vi "PiratiZKaribiku.vi"(11 "NXT/EV3":T1) -> (3 "NXT/EV3 2":T1)   [LabVIEW 2016]
uses:
  <vilib>/NXT/Subs/LVHSConnector.ctl
  <vilib>/NXT/LegoClasses/BrickReference/BrickReference.lvclass
  <vilib>/NXT/Dual Mode Library/Display/drawText_Center.vi
  <vilib>/NXT/Dual Mode Library/Sound/PlayA.vi
  <vilib>/NXT/Dual Mode Library/Sound/PlayC.vi
  <vilib>/NXT/Dual Mode Library/Sound/PlayD.vi
  <vilib>/NXT/Dual Mode Library/Sound/PlayE.vi
  <vilib>/NXT/Dual Mode Library/Sound/PlayF.vi
  <vilib>/NXT/Dual Mode Library/Sound/PlayG.vi
  <vilib>/NXT/Dual Mode Library/Waits/Wait_Num.vi
  <vilib>/NXT/Dual Mode Library/Sound/PlayB.vi
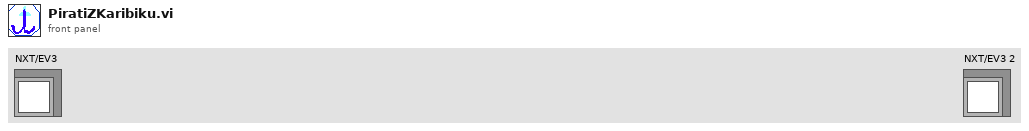
[diagram p1: front panel]
types:
  T1 = typedef "LVHSConnector.ctl" = refnum<class "BrickReference.lvclass">
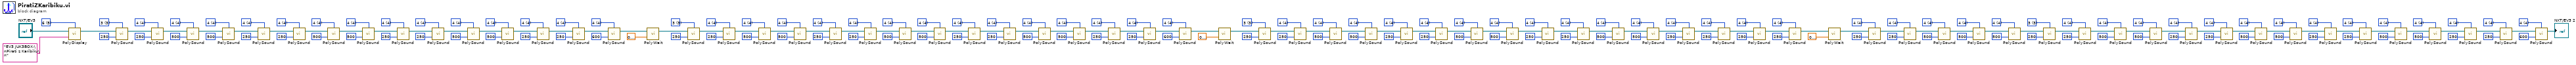
[diagram p0: block diagram]
diagram:
  w18 = u16 4 items=["3"=3, "4"=4, "5"=5, "6"=6, "7"=7] ("Octave")
  w21 = u16 4 items=["3"=3, "4"=4, "5"=5, "6"=6, "7"=7] ("Octave")
  w19 = u16 4 items=["3"=3, "4"=4, "5"=5, "6"=6, "7"=7] ("Octave")
  w26 = u16 4 items=["3"=3, "4"=4, "5"=5, "6"=6, "7"=7] ("Octave")
  w27 = u16 4 items=["3"=3, "4"=4, "5"=5, "6"=6, "7"=7] ("Octave")
  w28 = u16 4 items=["3"=3, "4"=4, "5"=5, "6"=6, "7"=7] ("Octave")
  w32 = u16 4 items=["3"=3, "4"=4, "5"=5, "6"=6, "7"=7] ("Octave")
  w33 = u16 4 items=["3"=3, "4"=4, "5"=5, "6"=6, "7"=7] ("Octave")
  w34 = u16 4 items=["3"=3, "4"=4, "5"=5, "6"=6, "7"=7] ("Octave")
  w36 = u16 4 items=["3"=3, "4"=4, "5"=5, "6"=6, "7"=7] ("Octave")
  w42 = u16 4 items=["3"=3, "4"=4, "5"=5, "6"=6, "7"=7] ("Octave")
  w43 = u16 4 items=["3"=3, "4"=4, "5"=5, "6"=6, "7"=7] ("Octave")
  w44 = u16 3 items=["3"=3, "4"=4, "5"=5, "6"=6, "7"=7] ("Octave")
  w45 = u16 4 items=["3"=3, "4"=4, "5"=5, "6"=6, "7"=7] ("Octave")
  w46 = u16 4 items=["3"=3, "4"=4, "5"=5, "6"=6, "7"=7] ("Octave")
  w49 = u16 4 items=["3"=3, "4"=4, "5"=5, "6"=6, "7"=7] ("Octave")
  w52 = u16 4 items=["3"=3, "4"=4, "5"=5, "6"=6, "7"=7] ("Octave")
  w55 = u16 4 items=["3"=3, "4"=4, "5"=5, "6"=6, "7"=7] ("Octave")
  w82 = u16 4 items=["3"=3, "4"=4, "5"=5, "6"=6, "7"=7] ("Octave")
  w83 = u16 4 items=["3"=3, "4"=4, "5"=5, "6"=6, "7"=7] ("Octave")
  w90 = u16 4 items=["3"=3, "4"=4, "5"=5, "6"=6, "7"=7] ("Octave")
  w89 = u16 4 items=["3"=3, "4"=4, "5"=5, "6"=6, "7"=7] ("Octave")
  w96 = u16 4 items=["3"=3, "4"=4, "5"=5, "6"=6, "7"=7] ("Octave")
  w97 = u16 4 items=["3"=3, "4"=4, "5"=5, "6"=6, "7"=7] ("Octave")
  w103 = u16 4 items=["3"=3, "4"=4, "5"=5, "6"=6, "7"=7] ("Octave")
  w100 = u16 4 items=["3"=3, "4"=4, "5"=5, "6"=6, "7"=7] ("Octave")
  w108 = u16 4 items=["3"=3, "4"=4, "5"=5, "6"=6, "7"=7] ("Octave")
  w107 = u16 4 items=["3"=3, "4"=4, "5"=5, "6"=6, "7"=7] ("Octave")
  w115 = u16 4 items=["3"=3, "4"=4, "5"=5, "6"=6, "7"=7] ("Octave")
  w119 = u16 4 items=["3"=3, "4"=4, "5"=5, "6"=6, "7"=7] ("Octave")
  w122 = u16 4 items=["3"=3, "4"=4, "5"=5, "6"=6, "7"=7] ("Octave")
  w129 = u16 4 items=["3"=3, "4"=4, "5"=5, "6"=6, "7"=7] ("Octave")
  w128 = u16 4 items=["3"=3, "4"=4, "5"=5, "6"=6, "7"=7] ("Octave")
  w127 = u16 3 items=["3"=3, "4"=4, "5"=5, "6"=6, "7"=7] ("Octave")
  w126 = u16 4 items=["3"=3, "4"=4, "5"=5, "6"=6, "7"=7] ("Octave")
  w125 = u16 4 items=["3"=3, "4"=4, "5"=5, "6"=6, "7"=7] ("Octave")
  w175 = u16 4 items=["3"=3, "4"=4, "5"=5, "6"=6, "7"=7] ("Octave")
  w169 = u16 4 items=["3"=3, "4"=4, "5"=5, "6"=6, "7"=7] ("Octave")
  w172 = u16 4 items=["3"=3, "4"=4, "5"=5, "6"=6, "7"=7] ("Octave")
  w164 = u16 4 items=["3"=3, "4"=4, "5"=5, "6"=6, "7"=7] ("Octave")
  w163 = u16 4 items=["3"=3, "4"=4, "5"=5, "6"=6, "7"=7] ("Octave")
  w162 = u16 4 items=["3"=3, "4"=4, "5"=5, "6"=6, "7"=7] ("Octave")
  w155 = u16 4 items=["3"=3, "4"=4, "5"=5, "6"=6, "7"=7] ("Octave")
  w154 = u16 4 items=["3"=3, "4"=4, "5"=5, "6"=6, "7"=7] ("Octave")
  w153 = u16 4 items=["3"=3, "4"=4, "5"=5, "6"=6, "7"=7] ("Octave")
  w150 = u16 4 items=["3"=3, "4"=4, "5"=5, "6"=6, "7"=7] ("Octave")
  w144 = u16 4 items=["3"=3, "4"=4, "5"=5, "6"=6, "7"=7] ("Octave")
  w143 = u16 4 items=["3"=3, "4"=4, "5"=5, "6"=6, "7"=7] ("Octave")
  w142 = u16 3 items=["3"=3, "4"=4, "5"=5, "6"=6, "7"=7] ("Octave")
  w141 = u16 4 items=["3"=3, "4"=4, "5"=5, "6"=6, "7"=7] ("Octave")
  w140 = u16 4 items=["3"=3, "4"=4, "5"=5, "6"=6, "7"=7] ("Octave")
  w178 = u16 4 items=["3"=3, "4"=4, "5"=5, "6"=6, "7"=7] ("Octave")
  w179 = i16 5 items=["1", "2", "3", "4", "5", "6", "7", "8", "9", "10", "11", "12"] ("Line")
  w183 = u16 4 items=["3"=3, "4"=4, "5"=5, "6"=6, "7"=7] ("Octave")
  w181 = u16 4 items=["3"=3, "4"=4, "5"=5, "6"=6, "7"=7] ("Octave")
  w188 = u16 4 items=["3"=3, "4"=4, "5"=5, "6"=6, "7"=7] ("Octave")
  w189 = u16 4 items=["3"=3, "4"=4, "5"=5, "6"=6, "7"=7] ("Octave")
  w190 = u16 4 items=["3"=3, "4"=4, "5"=5, "6"=6, "7"=7] ("Octave")
  w194 = u16 4 items=["3"=3, "4"=4, "5"=5, "6"=6, "7"=7] ("Octave")
  w195 = u16 4 items=["3"=3, "4"=4, "5"=5, "6"=6, "7"=7] ("Octave")
  w196 = u16 4 items=["3"=3, "4"=4, "5"=5, "6"=6, "7"=7] ("Octave")
  w198 = u16 4 items=["3"=3, "4"=4, "5"=5, "6"=6, "7"=7] ("Octave")
  w204 = u16 4 items=["3"=3, "4"=4, "5"=5, "6"=6, "7"=7] ("Octave")
  w205 = u16 4 items=["3"=3, "4"=4, "5"=5, "6"=6, "7"=7] ("Octave")
  w206 = u16 3 items=["3"=3, "4"=4, "5"=5, "6"=6, "7"=7] ("Octave")
  w207 = u16 4 items=["3"=3, "4"=4, "5"=5, "6"=6, "7"=7] ("Octave")
  w208 = u16 4 items=["3"=3, "4"=4, "5"=5, "6"=6, "7"=7] ("Octave")
  n1 = call-poly <vilib>:"PolyDisplay.vi"("Text"="EV3 JUK3BOX:\nPirati z Karibiku\n", "NXT/EV3"="NXT/EV3", "Line"=w179) -> ("NXT/EV3"=w78:T1)  [unwired: 1 in]
  n2 = call-poly <vilib>:"PolySound.vi"("Duration (500 ms)"=u16 250, "NXT/EV3"=w78, "Octave"=w206) -> ("NXT/EV3"=w77:T1)  [unwired: 1 in]
  n3 = call-poly <vilib>:"PolySound.vi"("Duration (500 ms)"=u16 250, "NXT/EV3"=w77, "Octave"=w208) -> ("NXT/EV3"=w76:T1)  [unwired: 1 in]
  n4 = call-poly <vilib>:"PolySound.vi"("Duration (500 ms)"=u16 500, "NXT/EV3"=w76, "Octave"=w207) -> ("NXT/EV3"=w75:T1)  [unwired: 1 in]
  n5 = call-poly <vilib>:"PolySound.vi"("Duration (500 ms)"=u16 500, "NXT/EV3"=w75, "Octave"=w205) -> ("NXT/EV3"=w74:T1)  [unwired: 1 in]
  n6 = call-poly <vilib>:"PolySound.vi"("Duration (500 ms)"=u16 250, "NXT/EV3"=w74, "Octave"=w204) -> ("NXT/EV3"=w73:T1)  [unwired: 1 in]
  n7 = call-poly <vilib>:"PolySound.vi"("Duration (500 ms)"=u16 250, "NXT/EV3"=w73, "Octave"=w198) -> ("NXT/EV3"=w72:T1)  [unwired: 1 in]
  n8 = call-poly <vilib>:"PolySound.vi"("Duration (500 ms)"=u16 500, "NXT/EV3"=w72, "Octave"=w196) -> ("NXT/EV3"=w71:T1)  [unwired: 1 in]
  n9 = call-poly <vilib>:"PolySound.vi"("Duration (500 ms)"=u16 500, "NXT/EV3"=w71, "Octave"=w195) -> ("NXT/EV3"=w70:T1)  [unwired: 1 in]
  n10 = call-poly <vilib>:"PolySound.vi"("Duration (500 ms)"=u16 250, "NXT/EV3"=w70, "Octave"=w194) -> ("NXT/EV3"=w69:T1)  [unwired: 1 in]
  n11 = call-poly <vilib>:"PolySound.vi"("Duration (500 ms)"=u16 250, "NXT/EV3"=w69, "Octave"=w190) -> ("NXT/EV3"=w68:T1)  [unwired: 1 in]
  n12 = call-poly <vilib>:"PolySound.vi"("Duration (500 ms)"=u16 500, "NXT/EV3"=w68, "Octave"=w188) -> ("NXT/EV3"=w67:T1)  [unwired: 1 in]
  n13 = call-poly <vilib>:"PolySound.vi"("Duration (500 ms)"=u16 500, "NXT/EV3"=w67, "Octave"=w189) -> ("NXT/EV3"=w66:T1)  [unwired: 1 in]
  n14 = call-poly <vilib>:"PolySound.vi"("Duration (500 ms)"=u16 250, "NXT/EV3"=w66, "Octave"=w181) -> ("NXT/EV3"=w65:T1)  [unwired: 1 in]
  n15 = call-poly <vilib>:"PolySound.vi"("Duration (500 ms)"=u16 250, "NXT/EV3"=w65, "Octave"=w183) -> ("NXT/EV3"=w64:T1)  [unwired: 1 in]
  n16 = call-poly <vilib>:"PolySound.vi"("Duration (500 ms)"=u16 600, "NXT/EV3"=w64, "Octave"=w178) -> ("NXT/EV3"=w63:T1)  [unwired: 1 in]
  n17 = call-poly <vilib>:"PolyWait.vi"("Time (1 sec)"=sgl 0.4, "NXT/EV3"=w63) -> ("NXT/EV3"=w139:T1)  [unwired: 2 in]
  n18 = call-poly <vilib>:"PolySound.vi"("Duration (500 ms)"=u16 250, "NXT/EV3"=w139, "Octave"=w142) -> ("NXT/EV3"=w62:T1)  [unwired: 1 in]
  n19 = call-poly <vilib>:"PolySound.vi"("Duration (500 ms)"=u16 250, "NXT/EV3"=w62, "Octave"=w140) -> ("NXT/EV3"=w61:T1)  [unwired: 1 in]
  n20 = call-poly <vilib>:"PolySound.vi"("Duration (500 ms)"=u16 500, "NXT/EV3"=w61, "Octave"=w141) -> ("NXT/EV3"=w60:T1)  [unwired: 1 in]
  n21 = call-poly <vilib>:"PolySound.vi"("Duration (500 ms)"=u16 500, "NXT/EV3"=w60, "Octave"=w143) -> ("NXT/EV3"=w59:T1)  [unwired: 1 in]
  n22 = call-poly <vilib>:"PolySound.vi"("Duration (500 ms)"=u16 250, "NXT/EV3"=w59, "Octave"=w144) -> ("NXT/EV3"=w58:T1)  [unwired: 1 in]
  n23 = call-poly <vilib>:"PolySound.vi"("Duration (500 ms)"=u16 250, "NXT/EV3"=w58, "Octave"=w150) -> ("NXT/EV3"=w57:T1)  [unwired: 1 in]
  n24 = call-poly <vilib>:"PolySound.vi"("Duration (500 ms)"=u16 500, "NXT/EV3"=w57, "Octave"=w153) -> ("NXT/EV3"=w56:T1)  [unwired: 1 in]
  n25 = call-poly <vilib>:"PolySound.vi"("Duration (500 ms)"=u16 500, "NXT/EV3"=w56, "Octave"=w154) -> ("NXT/EV3"=w152:T1)  [unwired: 1 in]
  n26 = call-poly <vilib>:"PolySound.vi"("Duration (500 ms)"=u16 250, "NXT/EV3"=w152, "Octave"=w155) -> ("NXT/EV3"=w159:T1)  [unwired: 1 in]
  n27 = call-poly <vilib>:"PolySound.vi"("Duration (500 ms)"=u16 250, "NXT/EV3"=w159, "Octave"=w162) -> ("NXT/EV3"=w160:T1)  [unwired: 1 in]
  n28 = call-poly <vilib>:"PolySound.vi"("Duration (500 ms)"=u16 500, "NXT/EV3"=w160, "Octave"=w164) -> ("NXT/EV3"=w161:T1)  [unwired: 1 in]
  n29 = call-poly <vilib>:"PolySound.vi"("Duration (500 ms)"=u16 500, "NXT/EV3"=w161, "Octave"=w163) -> ("NXT/EV3"=w173:T1)  [unwired: 1 in]
  n30 = call-poly <vilib>:"PolySound.vi"("Duration (500 ms)"=u16 250, "NXT/EV3"=w173, "Octave"=w172) -> ("NXT/EV3"=w170:T1)  [unwired: 1 in]
  n31 = call-poly <vilib>:"PolySound.vi"("Duration (500 ms)"=u16 250, "NXT/EV3"=w170, "Octave"=w169) -> ("NXT/EV3"=w174:T1)  [unwired: 1 in]
  n32 = call-poly <vilib>:"PolySound.vi"("Duration (500 ms)"=u16 600, "NXT/EV3"=w174, "Octave"=w175) -> ("NXT/EV3"=w112:T1)  [unwired: 1 in]
  n33 = call-poly <vilib>:"PolyWait.vi"("Time (1 sec)"=sgl 0.4, "NXT/EV3"=w112) -> ("NXT/EV3"=w111:T1)  [unwired: 2 in]
  n34 = call-poly <vilib>:"PolySound.vi"("Duration (500 ms)"=u16 250, "NXT/EV3"=w111, "Octave"=w127) -> ("NXT/EV3"=w131:T1)  [unwired: 1 in]
  n35 = call-poly <vilib>:"PolySound.vi"("Duration (500 ms)"=u16 250, "NXT/EV3"=w131, "Octave"=w125) -> ("NXT/EV3"=w123:T1)  [unwired: 1 in]
  n36 = call-poly <vilib>:"PolySound.vi"("Duration (500 ms)"=u16 500, "NXT/EV3"=w123, "Octave"=w126) -> ("NXT/EV3"=w130:T1)  [unwired: 1 in]
  n37 = call-poly <vilib>:"PolySound.vi"("Duration (500 ms)"=u16 500, "NXT/EV3"=w130, "Octave"=w128) -> ("NXT/EV3"=w124:T1)  [unwired: 1 in]
  n38 = call-poly <vilib>:"PolySound.vi"("Duration (500 ms)"=u16 250, "NXT/EV3"=w124, "Octave"=w129) -> ("NXT/EV3"=w120:T1)  [unwired: 1 in]
  n39 = call-poly <vilib>:"PolySound.vi"("Duration (500 ms)"=u16 250, "NXT/EV3"=w120, "Octave"=w122) -> ("NXT/EV3"=w117:T1)  [unwired: 1 in]
  n40 = call-poly <vilib>:"PolySound.vi"("Duration (500 ms)"=u16 500, "NXT/EV3"=w117, "Octave"=w119) -> ("NXT/EV3"=w114:T1)  [unwired: 1 in]
  n41 = call-poly <vilib>:"PolySound.vi"("Duration (500 ms)"=u16 500, "NXT/EV3"=w114, "Octave"=w115) -> ("NXT/EV3"=w105:T1)  [unwired: 1 in]
  n42 = call-poly <vilib>:"PolySound.vi"("Duration (500 ms)"=u16 250, "NXT/EV3"=w105, "Octave"=w107) -> ("NXT/EV3"=w110:T1)  [unwired: 1 in]
  n43 = call-poly <vilib>:"PolySound.vi"("Duration (500 ms)"=u16 250, "NXT/EV3"=w110, "Octave"=w108) -> ("NXT/EV3"=w99:T1)  [unwired: 1 in]
  n44 = call-poly <vilib>:"PolySound.vi"("Duration (500 ms)"=u16 500, "NXT/EV3"=w99, "Octave"=w100) -> ("NXT/EV3"=w104:T1)  [unwired: 1 in]
  n45 = call-poly <vilib>:"PolySound.vi"("Duration (500 ms)"=u16 500, "NXT/EV3"=w104, "Octave"=w103) -> ("NXT/EV3"=w93:T1)  [unwired: 1 in]
  n46 = call-poly <vilib>:"PolySound.vi"("Duration (500 ms)"=u16 250, "NXT/EV3"=w93, "Octave"=w97) -> ("NXT/EV3"=w94:T1)  [unwired: 1 in]
  n47 = call-poly <vilib>:"PolySound.vi"("Duration (500 ms)"=u16 250, "NXT/EV3"=w94, "Octave"=w96) -> ("NXT/EV3"=w87:T1)  [unwired: 1 in]
  n48 = call-poly <vilib>:"PolySound.vi"("Duration (500 ms)"=u16 250, "NXT/EV3"=w87, "Octave"=w89) -> ("NXT/EV3"=w92:T1)  [unwired: 1 in]
  n49 = call-poly <vilib>:"PolySound.vi"("Duration (500 ms)"=u16 250, "NXT/EV3"=w92, "Octave"=w90) -> ("NXT/EV3"=w86:T1)  [unwired: 1 in]
  n50 = call-poly <vilib>:"PolyWait.vi"("Time (1 sec)"=sgl 0.4, "NXT/EV3"=w86) -> ("NXT/EV3"=w79:T1)  [unwired: 2 in]
  n51 = call-poly <vilib>:"PolySound.vi"("Duration (500 ms)"=u16 250, "NXT/EV3"=w79, "Octave"=w83) -> ("NXT/EV3"=w80:T1)  [unwired: 1 in]
  n52 = call-poly <vilib>:"PolySound.vi"("Duration (500 ms)"=u16 250, "NXT/EV3"=w80, "Octave"=w82) -> ("NXT/EV3"=w50:T1)  [unwired: 1 in]
  n53 = call-poly <vilib>:"PolySound.vi"("Duration (500 ms)"=u16 500, "NXT/EV3"=w50, "Octave"=w55) -> ("NXT/EV3"=w51:T1)  [unwired: 1 in]
  n54 = call-poly <vilib>:"PolySound.vi"("Duration (500 ms)"=u16 500, "NXT/EV3"=w51, "Octave"=w52) -> ("NXT/EV3"=w47:T1)  [unwired: 1 in]
  n55 = call-poly <vilib>:"PolySound.vi"("Duration (500 ms)"=u16 500, "NXT/EV3"=w47, "Octave"=w49) -> ("NXT/EV3"=w2:T1)  [unwired: 1 in]
  n56 = call-poly <vilib>:"PolySound.vi"("Duration (500 ms)"=u16 250, "NXT/EV3"=w2, "Octave"=w44) -> ("NXT/EV3"=w16:T1)  [unwired: 1 in]
  n57 = call-poly <vilib>:"PolySound.vi"("Duration (500 ms)"=u16 250, "NXT/EV3"=w16, "Octave"=w46) -> ("NXT/EV3"=w15:T1)  [unwired: 1 in]
  n58 = call-poly <vilib>:"PolySound.vi"("Duration (500 ms)"=u16 500, "NXT/EV3"=w15, "Octave"=w45) -> ("NXT/EV3"=w14:T1)  [unwired: 1 in]
  n59 = call-poly <vilib>:"PolySound.vi"("Duration (500 ms)"=u16 500, "NXT/EV3"=w14, "Octave"=w43) -> ("NXT/EV3"=w13:T1)  [unwired: 1 in]
  n60 = call-poly <vilib>:"PolySound.vi"("Duration (500 ms)"=u16 250, "NXT/EV3"=w13, "Octave"=w42) -> ("NXT/EV3"=w12:T1)  [unwired: 1 in]
  n61 = call-poly <vilib>:"PolySound.vi"("Duration (500 ms)"=u16 250, "NXT/EV3"=w12, "Octave"=w36) -> ("NXT/EV3"=w11:T1)  [unwired: 1 in]
  n62 = call-poly <vilib>:"PolySound.vi"("Duration (500 ms)"=u16 500, "NXT/EV3"=w11, "Octave"=w34) -> ("NXT/EV3"=w10:T1)  [unwired: 1 in]
  n63 = call-poly <vilib>:"PolySound.vi"("Duration (500 ms)"=u16 500, "NXT/EV3"=w10, "Octave"=w33) -> ("NXT/EV3"=w9:T1)  [unwired: 1 in]
  n64 = call-poly <vilib>:"PolySound.vi"("Duration (500 ms)"=u16 250, "NXT/EV3"=w9, "Octave"=w32) -> ("NXT/EV3"=w8:T1)  [unwired: 1 in]
  n65 = call-poly <vilib>:"PolySound.vi"("Duration (500 ms)"=u16 250, "NXT/EV3"=w8, "Octave"=w28) -> ("NXT/EV3"=w7:T1)  [unwired: 1 in]
  n66 = call-poly <vilib>:"PolySound.vi"("Duration (500 ms)"=u16 500, "NXT/EV3"=w7, "Octave"=w26) -> ("NXT/EV3"=w6:T1)  [unwired: 1 in]
  n67 = call-poly <vilib>:"PolySound.vi"("Duration (500 ms)"=u16 500, "NXT/EV3"=w6, "Octave"=w27) -> ("NXT/EV3"=w5:T1)  [unwired: 1 in]
  n68 = call-poly <vilib>:"PolySound.vi"("Duration (500 ms)"=u16 250, "NXT/EV3"=w5, "Octave"=w19) -> ("NXT/EV3"=w4:T1)  [unwired: 1 in]
  n69 = call-poly <vilib>:"PolySound.vi"("Duration (500 ms)"=u16 250, "NXT/EV3"=w4, "Octave"=w21) -> ("NXT/EV3"=w3:T1)  [unwired: 1 in]
  n70 = call-poly <vilib>:"PolySound.vi"("Duration (500 ms)"=u16 600, "NXT/EV3"=w3, "Octave"=w18) -> ("NXT/EV3"=→"NXT/EV3 2":T1)  [unwired: 1 in]
